vi "SS Generate Device String.vi"(8 "error in (no error)":errorcluster, 10 "Suffix":string, 11 "Info":T1={"Type"="", "Model"="", "Ch Names"=[], "Ch Units"=[], "Channel Data"=[], "Status"={"Status"=enum."Initializing", "Data"=variant}, "Address"=""}) -> (0 "error out":errorcluster, 3 "output string":string)   [LabVIEW 2021]
uses:
  SS typedef cluster Instrument Cmd Q Device Info Response.ctl
  SS enum Channel Data Type.ctl
  SS cluster Status.ctl
  SS enum Status.ctl
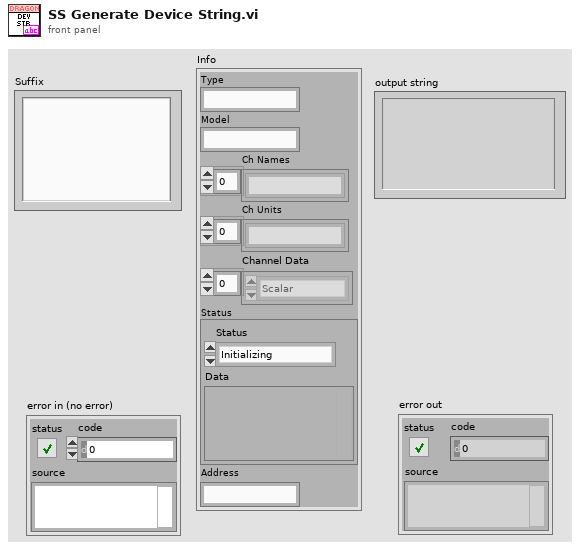
[diagram p1: front panel]
types:
  T1 = typedef "SS typedef cluster Instrument Cmd Q Device Info Response.ctl" = cluster{"Type":string, "Model":string, "Ch Names":string[], "Ch Units":string[], "Channel Data":T2[], "Status":T3, "Address":string}
  T2 = typedef "SS enum Channel Data Type.ctl" = enum16{"Scalar", "Waveform", "Text", "Other"}
  T3 = typedef "SS cluster Status.ctl" = cluster{"Status":T4, "Data":variant}
  T4 = typedef "SS enum Status.ctl" = enum16{"Unknown", "Running", "Initializing", "Idle", "Error"}
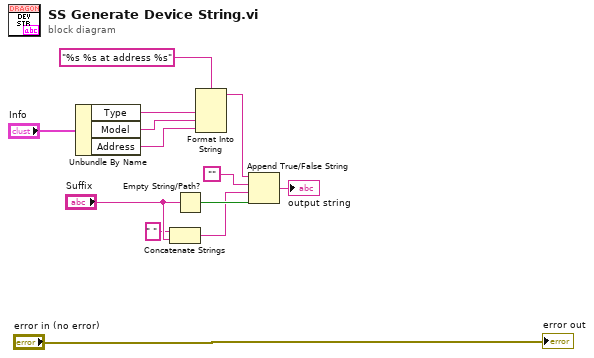
[diagram p0: block diagram]
diagram:
  n1 = Unbundle By Name("Info") -> ("Type"=w10:string, "Model"=w9:string, "Address"=w8:string)
  n2 = Concatenate Strings(" " ("string"), "Suffix") -> (w1:string)
  n3 = Empty String/Path?(string/path="Suffix") -> (empty?=w6:bool)
  n4 = Format Into String(format string="%s %s at address %s", w10, w9, w8) -> (resulting string=w7:string)  [unwired: 2 in, 1 out]
  n5 = Append True/False String(1:w6, 2:w1, 3:"", 4:w7) -> (0:→"output string":string)
  "error out" <- "error in (no error)"
